vi "Write algoparameters JSON.vi"(0 "JSON FilePath":path=path "F:/Backup/ZenGage v3.0/20-02-2018/ZenGage v1.1/Configuration file/Algorithm Override JSON.json", 1 "Part Name":string="102", 2 "Algo override variant":variant, 5 "Input data cluster":T1={"Tolerance Limits"=[[0.0, 1.0, 0.0, 1.0]], "Measurement Enable"=[TRUE], "Bias Correction"=[0.1], "Linearity Correction"=[0.2], "Measurement names"=[]}, 7 "Variant":bool, 9 "Ticked measurements":i32[](array[numeric])=[0], 11 "error in (no error)":errorcluster, 12 "User interface enqueuer":refnum<class "Message Enqueuer.lvclass">) -> (4 "JSON Variant":variant, 15 "error out":errorcluster)   [LabVIEW 2019, in "ZenGage v3.0 UI.lvclass"]
uses:
  ZenGage v3.0 UI.lvclass
  User Interface Messages/User Interface messages/Display Popup Msg/DisplayPopup_UI.lvclass
  Common/Controls/Pop-up Input.ctl
  <vilib>/ActorFramework/Message Enqueuer/Message Enqueuer.lvclass
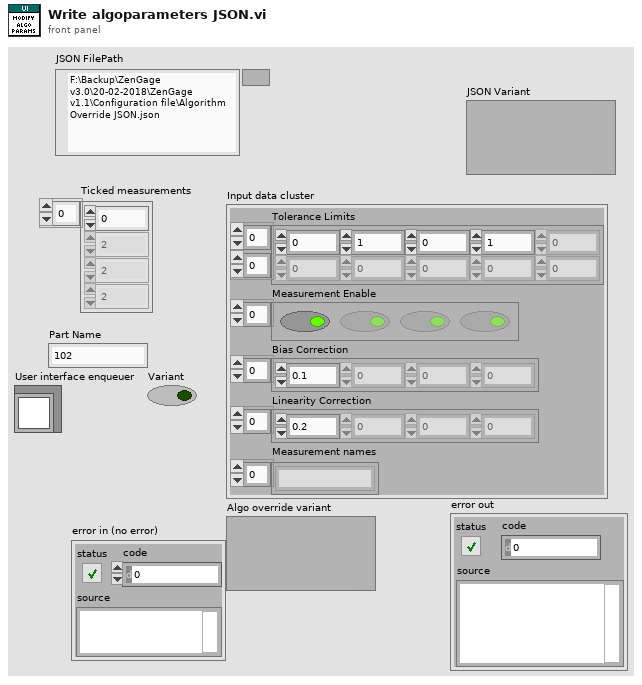
[diagram p1: front panel]
types:
  T1 = cluster{"Tolerance Limits":dbl[][], "Measurement Enable":bool[], "Bias Correction":dbl[], "Linearity Correction":dbl[], "Measurement names":string[]}
  T2 = enum16{"Open Logo Display", "Close Logo Display", "Open Loading Bar", "Close Loading Bar", "Open Alert Display", "Close Alert Display", "One button dialog box", "Two button dialog box", "User Authentication"}
  T3 = typedef "Pop-up Input.ctl" = cluster{"Pop-up Type":enum16{"Open Logo Display", "Close Logo Display", "Open Loading Bar", "Close Loading Bar", "Open Alert Display", "Close Alert Display", "One button dialog box", "Two button dialog box", "User Authentication"}, "Title":string, "Message":string, "Button 1 Text":string, "Button 2 Text":string, "Show Close? T/F":bool, "Title Blink? T/F":bool, "Title Blink Colour":u32}
  T4 = enum16{"Action Failed", "Append", "Insert", "Replace"}
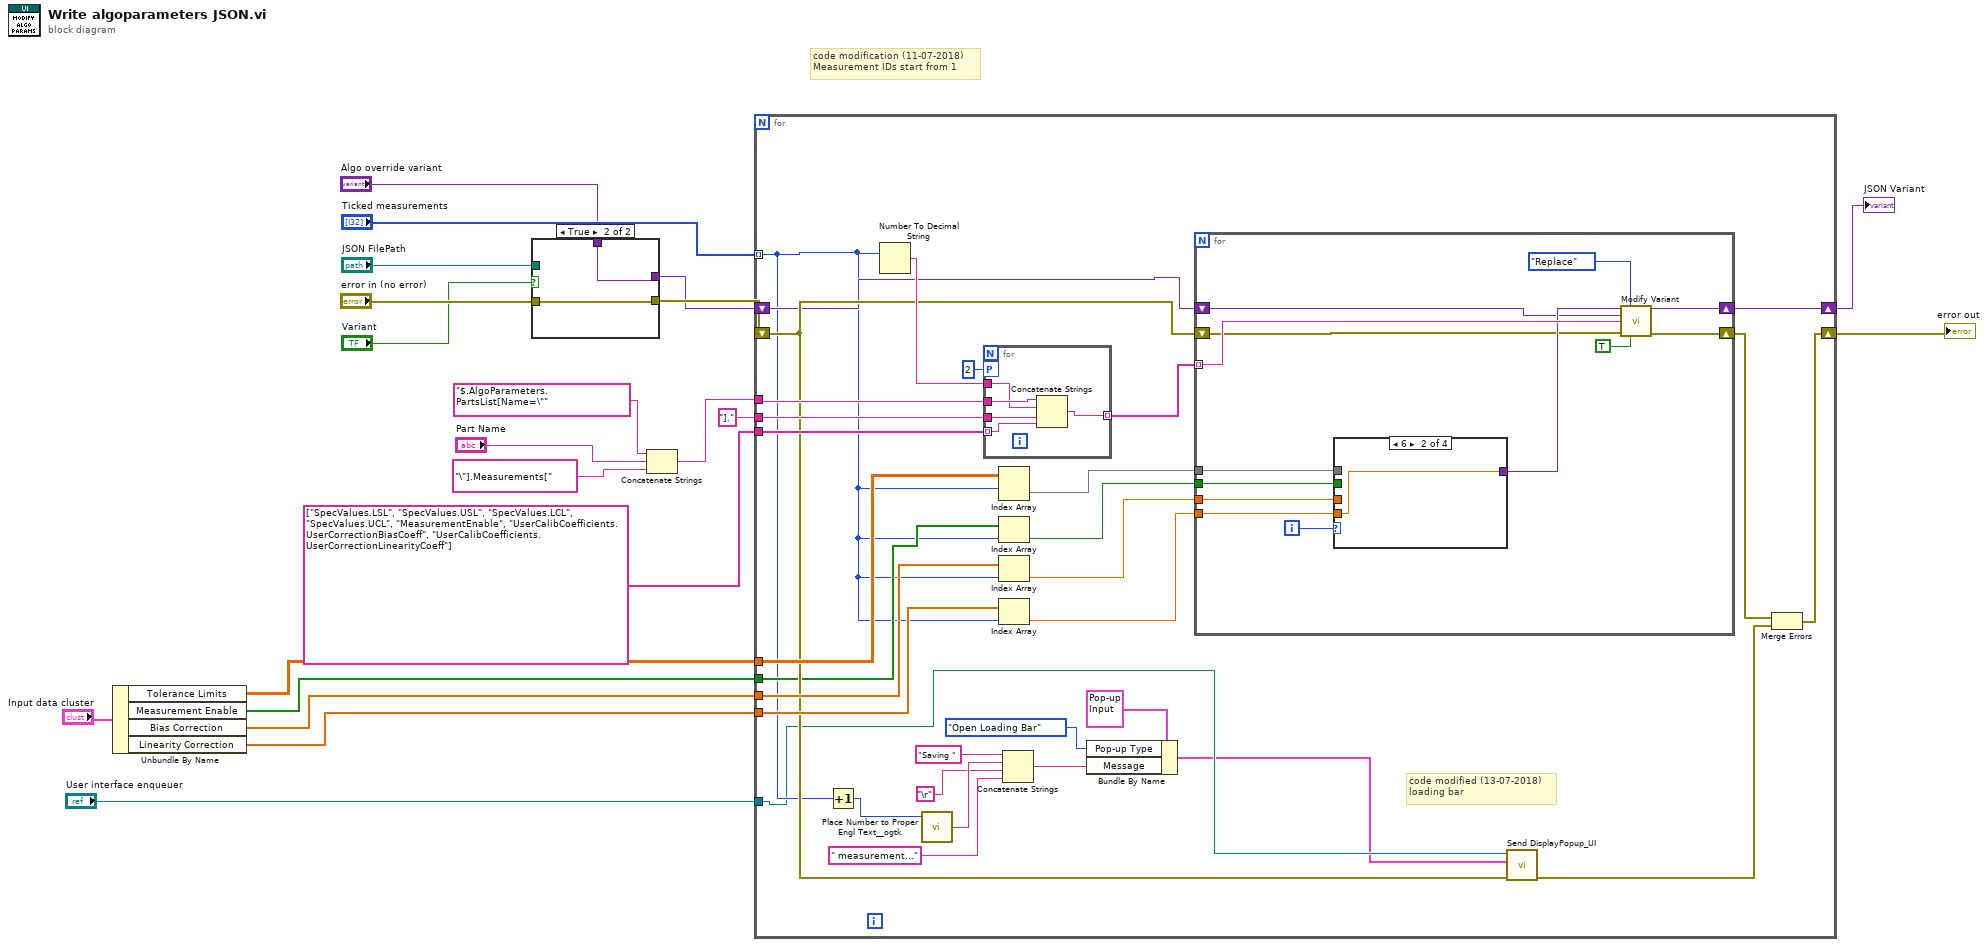
[diagram p0: block diagram]
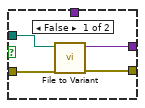
[diagram p2: hidden frame]
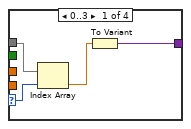
[diagram p3: hidden frame]
diagram:
  # "code modification (11-07-2018)\nMeasurement IDs start from 1"
  n1 = Unbundle By Name("Input data cluster") -> ("Tolerance Limits"=w10:dbl[][], "Measurement Enable"=w9:bool[], "Bias Correction"=w8:dbl[], "Linearity Correction"=w7:dbl[])
  n2 = case shown="True" "Variant" {
    tunnel: "error in (no error)" -> [w25 w26]
    tunnel: [w24 w26] -> w19
    tunnel: "JSON FilePath" -> [w23 _]
    tunnel: [w22 w27] -> w17
    tunnel: "Algo override variant" -> [_ w27]
    frame False {
      n3 = call <vilib>:"File to Variant.vi"("JSON FilePath"=w23, "error in (no error)"=w25) -> ("JSON Variant"=w22:variant, "error out"=w24:errorcluster)  [unwired: 6 in, 1 out]
    }
    frame True {
    }
  }
  n4 = Concatenate Strings("$.AlgoParameters.PartsList[Name=\"", "Part Name", "\"].Measurements[") -> (w12:string)
  n5 = for {
    tunnel: "Ticked measurements" -> [w37] mode=indexing
    shift-right: [w33] -> w4
    shift-left: w19 -> [w45]
    tunnel: w12 -> [w58]
    tunnel: string[] ["SpecValues.LSL", "SpecValues.USL", "SpecValues.LCL", "SpecValues.UCL", "MeasurementEnable", "UserCalibCoefficients.UserCorrectionBiasCoeff", "UserCalibCoefficients.UserCorrectionLinearityCoeff"] -> [w57]
    shift-right: [w55] -> w6
    shift-left: w17 -> [w44]
    tunnel: w10 -> [w54]
    tunnel: w9 -> [w43]
    tunnel: w8 -> [w51]
    tunnel: w7 -> [w50]
    tunnel: "]." ("string") -> [w47]
    tunnel: "User interface enqueuer" -> [w32]
    # "code modified (13-07-2018)\nloading bar"
    n6 = Increment(x=w37) -> (x+1=w36:i32)
    n7 = Number To Decimal String(number=w37) -> (decimal integer string=w46:string)  [unwired: 1 in]
    n8 = call <userlib>:"Place Number to Proper Engl Text__ogtk.vi"("Numeric"=w36) -> ("String"=w40:string)  [unwired: 4 in]
    n9 = for {
      tunnel: w58 -> [w63]
      tunnel: w46 -> [w62]
      tunnel: w57 -> [w60] mode=indexing
      tunnel: [w61] -> w56 mode=indexing
      tunnel: w47 -> [w59]
      workers-P: 2 -> [_]
      n10 = Concatenate Strings(w63, w62, w59, w60) -> (w61:string)
    }
    n11 = Index Array(array=w54, index (row)=w37) -> (element=w53:dbl[])  [unwired: 1 in]
    n12 = Index Array(array=w43, index=w37) -> (element=w52:bool)
    n13 = Index Array(array=w51, index=w37) -> (element=w49:dbl)
    n14 = Index Array(array=w50, index=w37) -> (element=w48:dbl)
    n15 = Concatenate Strings("Saving " ("string"), w40, "\r", " measurement..." ("string")) -> (w38:string)
    n16 = Bundle By Name(cluster=T3 {"Pop-up Type"=enum."Open Logo Display", "Title"="", "Message"="", "Button 1 Text"="", "Button 2 Text"="", "Show Close? T/F"=FALSE, "Title Blink? T/F"=FALSE, "Title Blink Colour"=0} ("PopupDetails"), "Pop-up Type"=T2."Open Loading Bar", "Message"=w38) -> (w30:T3)
    n17 = for {
      shift-right: [w65] -> w34
      shift-left: w45 -> [w66]
      tunnel: w56 -> [w76] mode=indexing
      shift-right: [w74] -> w55
      shift-left: w44 -> [w67]
      tunnel: w53 -> [w68]
      tunnel: w52 -> [w71]
      tunnel: w49 -> [w70]
      tunnel: w48 -> [w69]
      i -> [w73]
      n18 = case shown="6" w73 {
        selector: w73 -> [w79 _ _ _]
        tunnel: w68 -> [w78 _ _ _]
        tunnel: [w80 w81 w82 w83] -> w72
        tunnel: w71 -> [_ _ w82 _]
        tunnel: w70 -> [_ _ _ w83]
        tunnel: w69 -> [_ w81 _ _]
        frame 0..3 {
          n19 = Index Array(array=w78, index=w79) -> (element=w77:dbl)
          n20 = To Variant(anything=w77) -> (Variant=w80:variant)
        }
        frame 6 {
        }
        frame 4, Default {
        }
        frame 5 {
        }
      }
      n21 = call <vilib>:"Modify Variant.vi"("New element in"=w72, "Functionality"=T4."Replace", "Parent variant in"=w67, "JSON query path"=w76, "error in (no error)"=w66, "Overwrite\n(Ignore datatype?)"=TRUE ("Overwrite\n(Ignore datatype?)")) -> ("VCluster out"=w74:variant, "error out"=w65:errorcluster)  [unwired: 5 in, 3 out]
    }
    n22 = call "Send DisplayPopup_UI.vi"("error in (no error)"=w45, "PopupDetails"=w30, "Message Enqueuer"=w32) -> ("error out"=w35:errorcluster)  [unwired: 7 in, 1 out]
    n23 = Merge Errors(w34, w35) -> (w33:errorcluster)
  }
  "JSON Variant" <- w6
  "error out" <- w4
